vi "Edit_Template_File.vi"(0 "Mode":T3(ring), 7 "Template Filename":path, 11 "Data Filename":path) -> (6 "Template Filename Out":path)   [LabVIEW 2016]
uses:
  Anemometry/Anemometry Sub Vis/Data_plotting_vis/File_Template_Clus.ctl
  subVIs/Dispose_Channel.ctl
  Anemometry/Anemometry Sub Vis/Controls/Global_mode.ctl
panel:
  out "index of element":i32
  in  "Add New Channel Named":bool
  in  "Edit Maths Equation":bool
  out "Current Case Name":string
  in  "Organise Channels":bool
  in  "Add New Channels Fr File":bool
  in  "OK":bool
  in  "Search String":string
  in  "Listbox":i32(listbox)
  out "Channel Name":string
  in  "Cluster":T1 {"Tolerance" min=0.0 format="%#.4f"}
  # "> 20  or  <20  or  =hello   or \n£hello  (not equal to hello)"
  # "<<Characters_to_Match>>  <<Replace_Whole_String_with_this>>"
  # "<<Channel_Name>> contains <<Characters to match>> or\n<<Channel_Name>> does not contain <<Characters to match>>"
  # "<<Channel_Name_A>> + <<Channel_Name_B>> or\nConcatenate <<Channel_Name_A>> and <<Channel_Name_B>>"
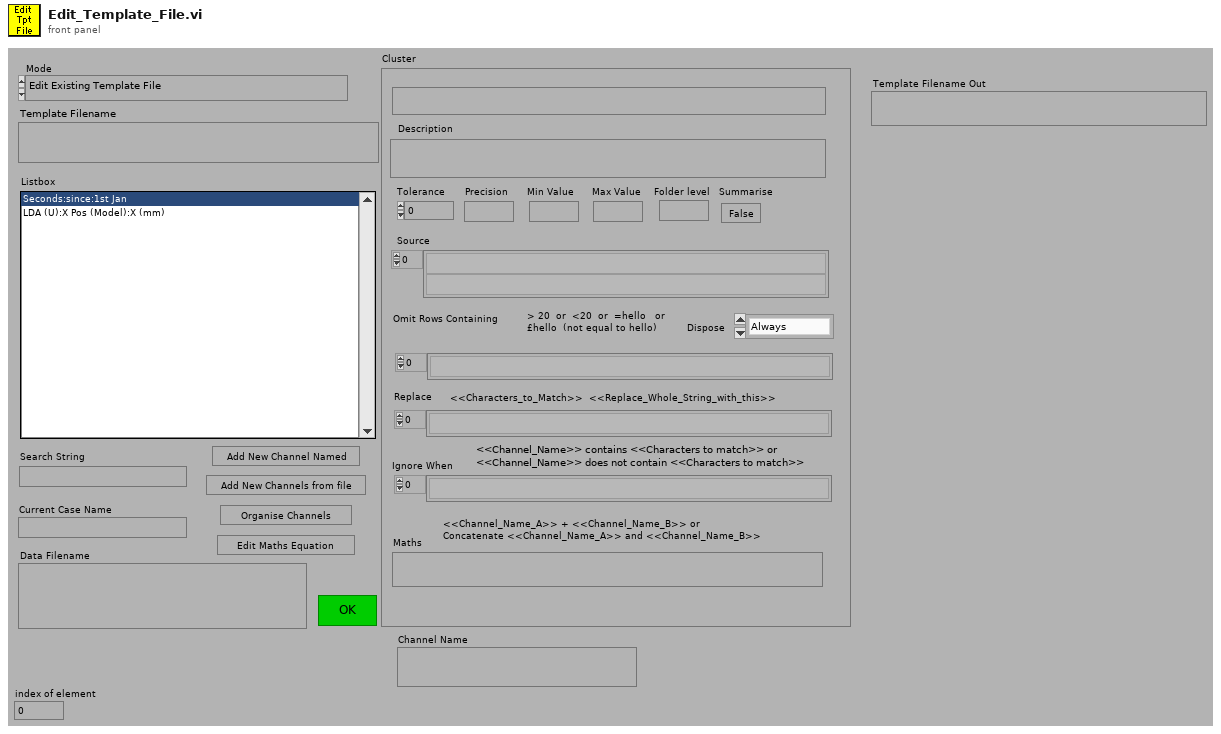
[diagram p1: front panel]
types:
  T1 = typedef "File_Template_Clus.ctl" = cluster{"Template Channel Name":string, "Description":string, "Tolerance":dbl, "Precision":string, "Folder level":string, "Source":string[], "Replace":string[], "Summarise":bool, "Min Value":string, "Maths":string, "Omit Rows Containing":string[], "Ignore When":string[], "Max Value":string, "Dispose":T2}
  T2 = typedef "Dispose_Channel.ctl" = enum16{"Always", "If Blank", "Never"}
  T3 = enum16{"Edit Existing Template File", "Create New Template File"}
  T4 = typedef "Global_mode.ctl" = enum16{"Read Global", "Load Global From File", "Write Global to File"}
  T5 = enum16{"Read Channels From File", "Read Channels from Server"}
  T6 = enum32{"existing file", "new file", "new or existing file", "existing dir", "new dir", "new or existing dir", "existing file (use LLBs)", "new file (use LLBs)", "new or existing file (use LLBs)", "new or existing file or directory (use LLBs)"}
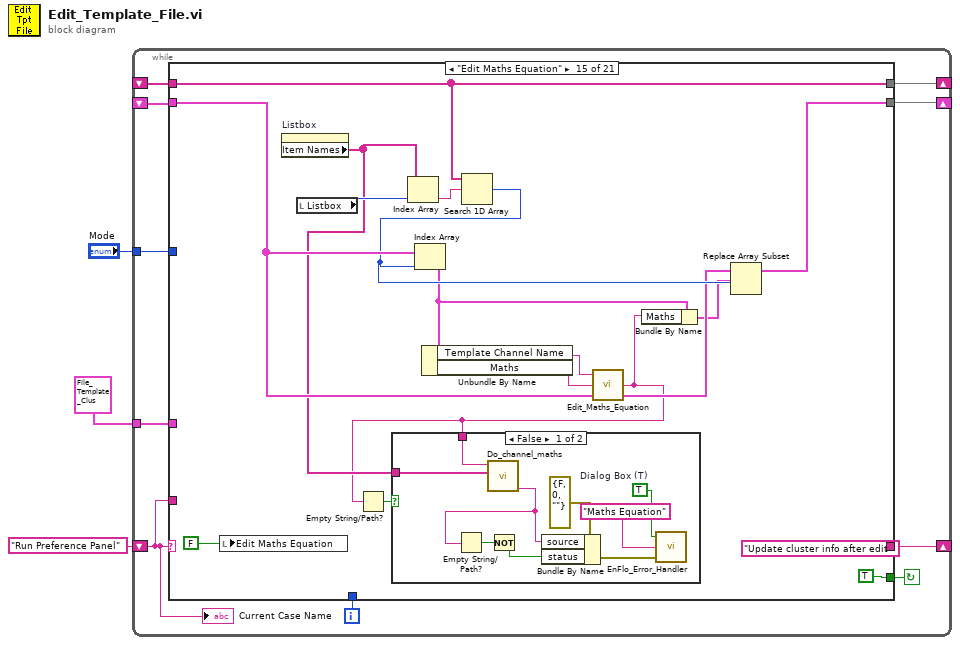
[diagram p0: block diagram]
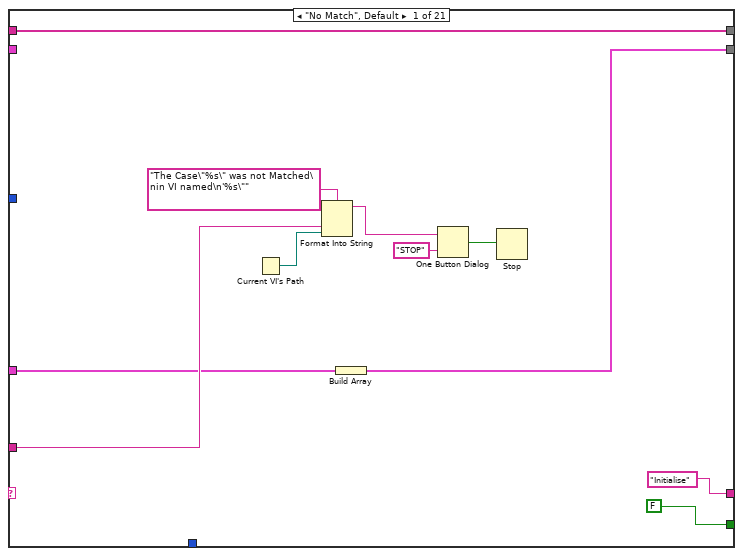
[diagram p2: hidden frame]
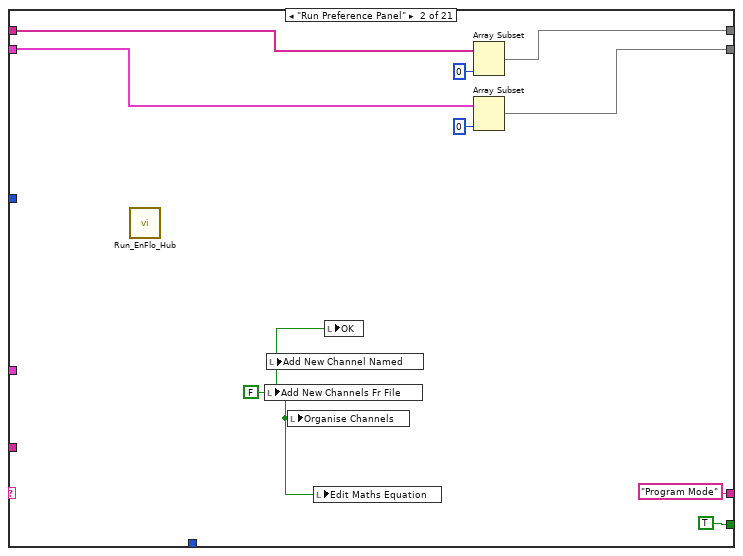
[diagram p3: hidden frame]
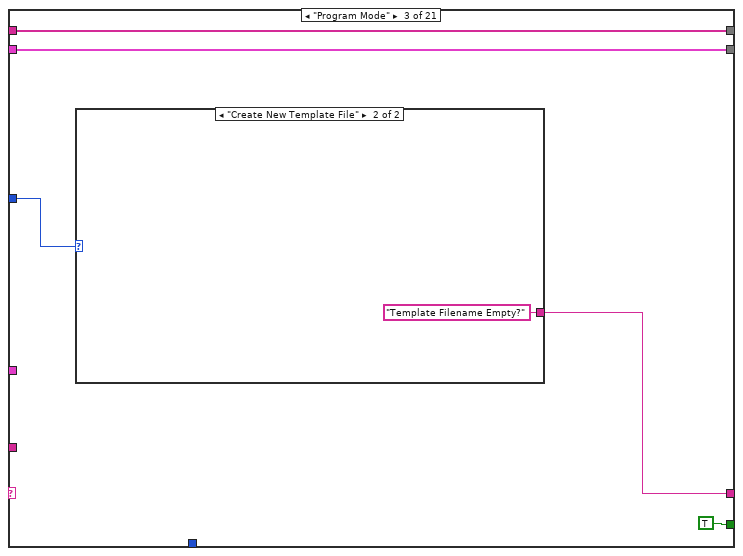
[diagram p4: hidden frame]
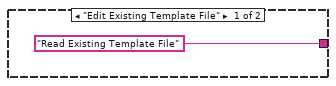
[diagram p5: hidden frame]
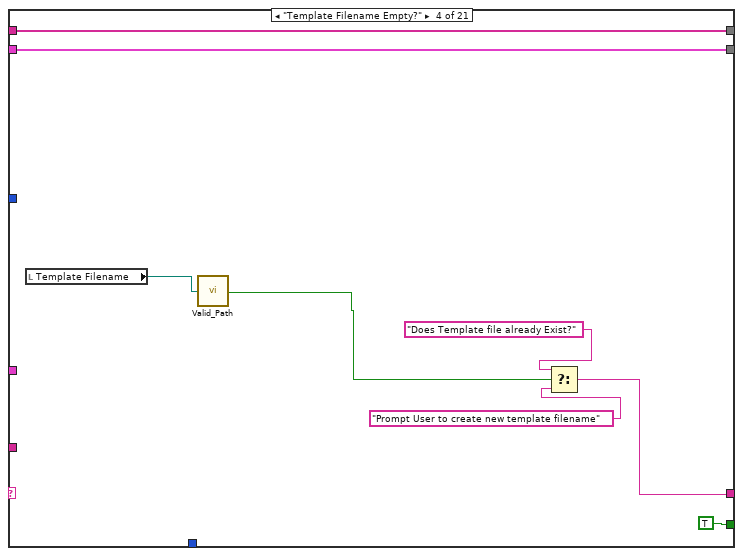
[diagram p6: hidden frame]
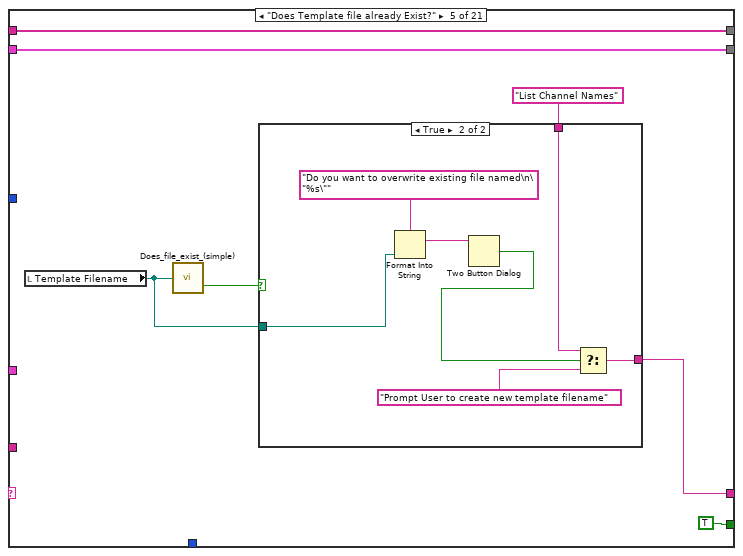
[diagram p7: hidden frame]
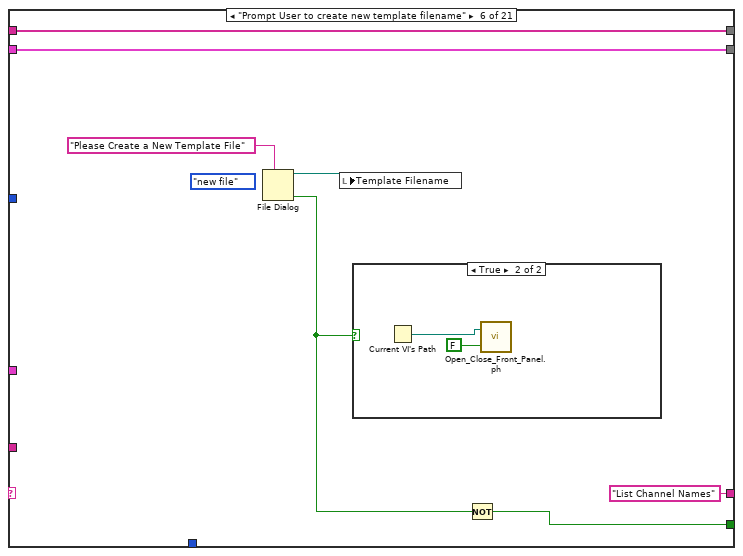
[diagram p9: hidden frame]
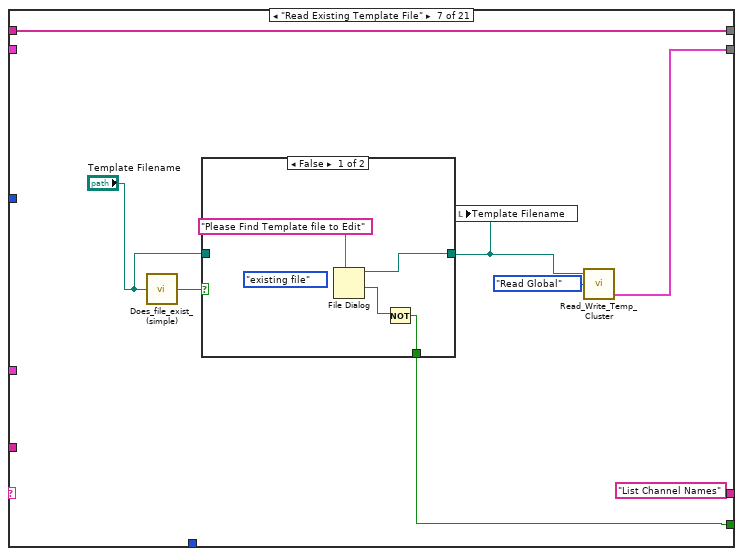
[diagram p11: hidden frame]
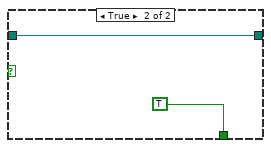
[diagram p12: hidden frame]
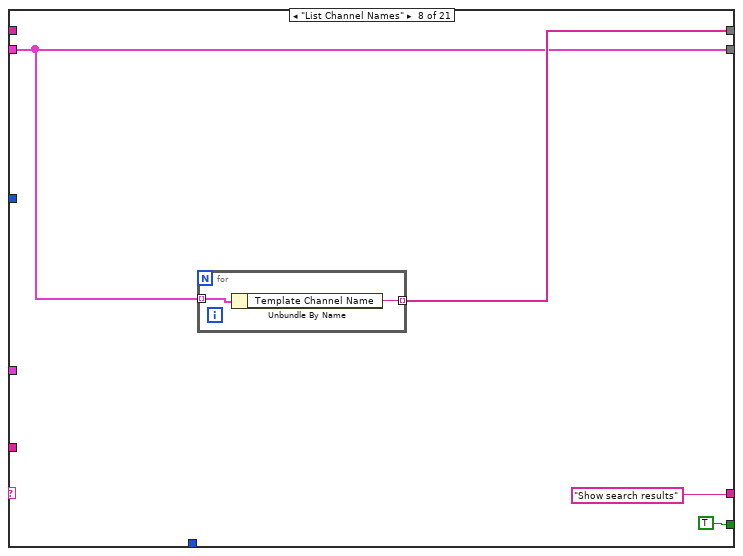
[diagram p13: hidden frame]
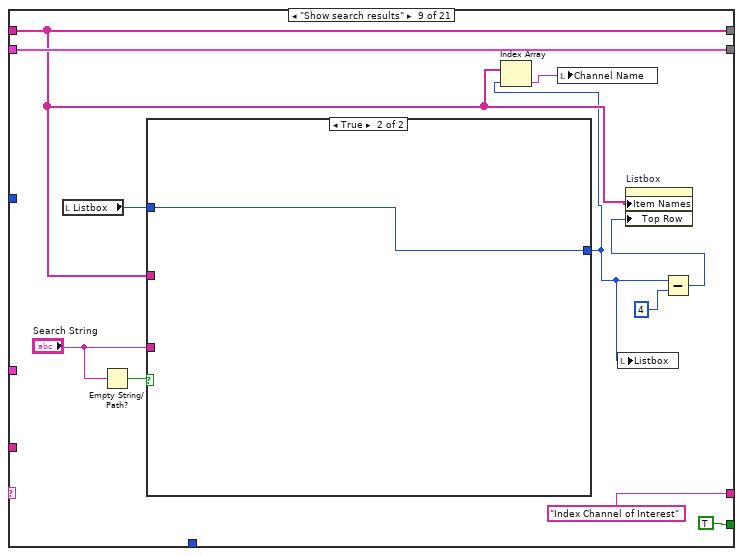
[diagram p14: hidden frame]
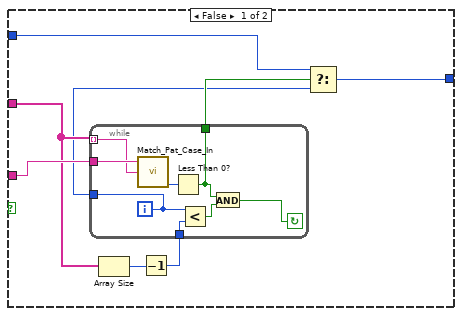
[diagram p15: hidden frame]
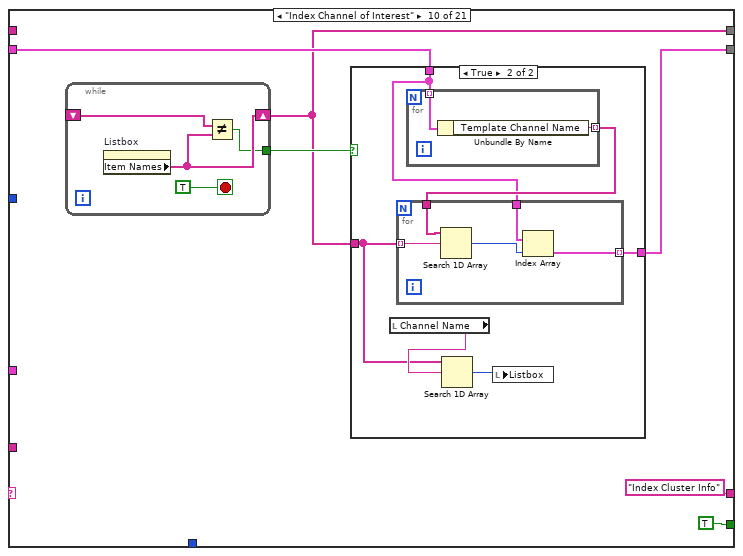
[diagram p16: hidden frame]
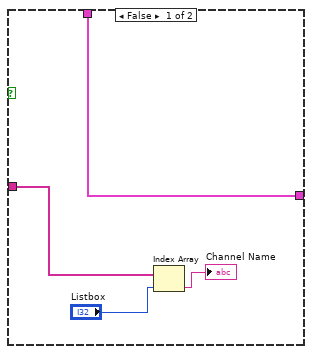
[diagram p17: hidden frame]
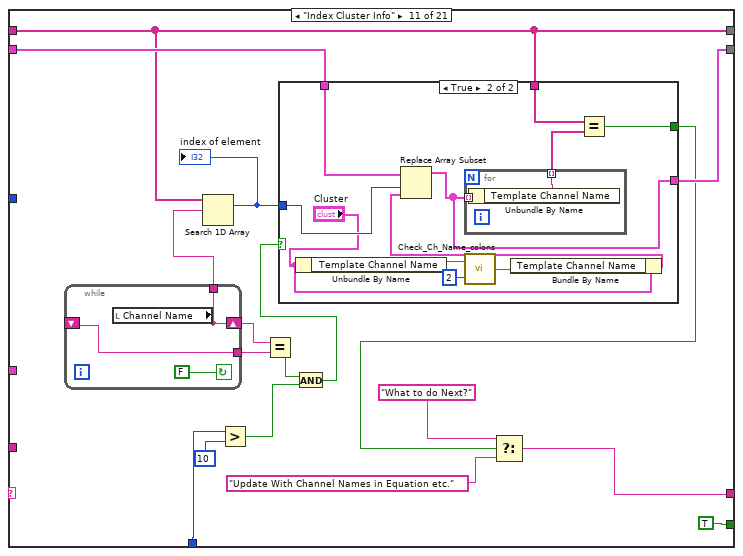
[diagram p18: hidden frame]
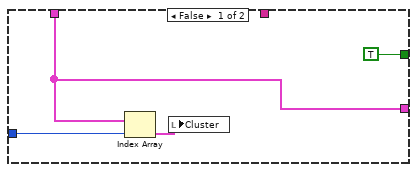
[diagram p19: hidden frame]
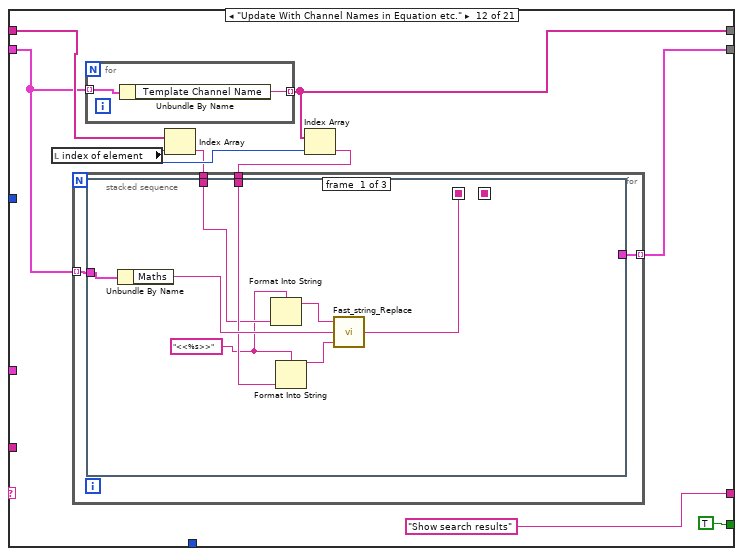
[diagram p20: hidden frame]
diagram:
  n1 = while {
    tunnel: T1 {"Template Channel Name"="", "Description"="", "Tolerance"=0.0, "Precision"="", "Folder level"="", "Source"=[], "Replace"=[], "Summarise"=FALSE, "Min Value"="", "Maths"="", "Omit Rows Containing"=[], "Ignore When"=[], "Max Value"="", "Dispose"=enum."Never"} ("Cluster") -> [w7]
    shift-left: _ -> [w8]
    shift-right: [w9] -> _
    tunnel: "Mode" -> [w11]
    shift-left: _ -> [w4]
    shift-right: [w10] -> _
    shift-left: "Run Preference Panel" -> [w6]
    shift-right: [w12] -> _
    i -> [w5]
    stop <- w13 continue-if-true
    n2 = case shown="\"Edit Maths Equation\"" w6 {
      tunnel: [FALSE TRUE TRUE TRUE TRUE w65 w73 TRUE TRUE TRUE TRUE TRUE TRUE TRUE TRUE TRUE TRUE TRUE TRUE TRUE FALSE] -> w13
      tunnel: ["Initialise" "Program Mode" w34 w45 w50 "List Channel Names" ("t") "List Channel Names" "Show search results" "Index Channel of Interest" "Index Cluster Info" w155 "Show search results" "Update cluster info after edit" "Update cluster info after edit" "Update cluster info after edit" "Save Template File" ("t") w333 w342 "Save Template File" w371 "End" ("t")] -> w12
      tunnel: w6 -> [w19 _ _ _ _ _ _ _ _ _ _ _ _ _ _ _ _ _ _ _ _]
      tunnel: w11 -> [_ _ w37 _ _ _ _ _ _ _ _ _ _ _ _ _ _ _ _ _ _]
      tunnel: [w14 w26 w35 w46 w53 w69 w76 w87 w99 w123 w158 w190 w228 w270 w287 w311 w336 w348 w362 w376 w383] -> w10
      tunnel: w4 -> [_ w27 w35 w46 w53 w69 _ w87 w99 w124 w162 w189 w230 w271 w292 w311 w336 w349 w368 w376 w383]
      tunnel: [w16 w29 w36 w47 w54 w70 w75 w89 w95 w121 w154 w191 w229 w272 w294 w313 w337 w350 w363 w375 w384] -> w9
      tunnel: w8 -> [w16 w30 w36 w47 w54 w70 w75 _ w95 _ w154 w192 w231 w273 w294 w313 w337 w350 w364 w375 w384]
      tunnel: w7 -> [w15 _ _ _ _ _ _ _ _ _ _ _ w227 _ _ _ _ _ w367 _ _]
      tunnel: w5 -> [_ _ _ _ _ _ _ _ _ _ w152 _ _ _ _ _ _ _ _ _ _]
      frame "No Match", Default {
        n3 = Current VI's Path() -> (path=w18:path)
        n4 = Format Into String(format string="The Case\"%s\" was not Matched\nin VI named\n'%s\"" ("Format String"), w19, w18) -> (resulting string=w22:string)  [unwired: 2 in, 1 out]
        n5 = Build Array(w15) -> (w14:T1[])
        n6 = One Button Dialog(message=w22, button name ("OK")="STOP") -> (true=w20:bool)
        n7 = Stop(stop? (T)=w20) -> ()
      }
      frame "Run Preference Panel" {
        w25 = FALSE ("Add channel Fr Results File")
        n8 = call "Run_EnFlo_Hub.vi"() -> ()  [unwired: 1 in, 7 out]
        n9 = local write "Add New Channels Fr File"(w25) -> ()
        n10 = local write "Add New Channel Named"(w25) -> ()
        n11 = local write "Organise Channels"(w25) -> ()
        n12 = local write "Edit Maths Equation"(w25) -> ()
        n13 = local write "OK"(w25) -> ()
        n14 = Array Subset(array=w30, length=0 ("Array Length")) -> (w29:string[])  [unwired: 1 in]
        n15 = Array Subset(array=w27, length=0 ("Array Length")) -> (w26:T1[])  [unwired: 1 in]
      }
      frame "Program Mode" {
        n16 = case shown="\"Create New Template File\"" w37 {
          tunnel: ["Read Existing Template File" "Template Filename Empty?"] -> w34
          frame "Edit Existing Template File" {
          }
          frame "Create New Template File" {
          }
        }
      }
      frame "Template Filename Empty?" {
        n17 = local read "Template Filename"() -> (w44:path)
        n18 = call "Valid_Path.vi"("Filename"=w44) -> ("Valid Path?"=w43:bool)
        n19 = Select(t="Does Template file already Exist?", s=w43, f="Prompt User to create new template filename" ("t")) -> (s? t:f=w45:string)
      }
      frame "Does Template file already Exist?" {
        n20 = local read "Template Filename"() -> (w51:path)
        n21 = call "Does_file_exist_(simple).vi"("Pathname"=w51) -> ("exists?"=w52:bool)
        n22 = case shown="True" w52 {
          tunnel: w51 -> [_ w63]
          tunnel: [w56 w58] -> w50
          tunnel: "List Channel Names" ("t") -> [w56 w57]
          frame False {
          }
          frame True {
            n23 = Format Into String(format string="Do you want to overwrite existing file named\n\"%s\"" ("Format String"), w63) -> (resulting string=w61:string)  [unwired: 2 in, 1 out]
            n24 = Two Button Dialog(message=w61) -> (T button?=w59:bool)  [unwired: 2 out]
            n25 = Select(t=w57, s=w59, f="Prompt User to create new template filename") -> (s? t:f=w58:string)
          }
        }
      }
      frame "Prompt User to create new template filename" {
        (unwired) T6."new file" ("select mode (2)")
        n26 = File Dialog(7:"Please Create a New Template File" ("prompt")) -> (1:w64:bool, 3:w68:path)  [unwired: 1 in, 7 out]
        n27 = local write "Template Filename"(w68) -> ()
        n28 = case shown="True" w64 {
          frame False {
          }
          frame True {
            n29 = Current VI's Path() -> (path=w72:path)
            n30 = call "Open_Close_Front_Panel.ph.vi"("Front Panel Window:Open"=FALSE, "VI path"=w72) -> ()  [unwired: 2 out]
          }
        }
        n31 = Not(x=w64) -> (.not. x?=w65:bool)
      }
      frame "Read Existing Template File" {
        n32 = call "Does_file_exist_(simple).vi"("Pathname"="Template Filename") -> ("exists?"=w79:bool)
        n33 = case shown="False" w79 {
          tunnel: [w84 w86] -> w74
          tunnel: "Template Filename" -> [_ w86]
          tunnel: [w81 TRUE] -> w73
          frame False {
            (unwired) T6."existing file" ("select mode (2)")
            n34 = File Dialog(7:"Please Find Template file to Edit" ("prompt")) -> (1:w82:bool, 3:w84:path)  [unwired: 1 in, 7 out]
            n35 = Not(x=w82) -> (.not. x?=w81:bool)
          }
          frame True {
          }
        }
        n36 = local write "Template Filename"(w74) -> ()
        n37 = call "Read_Write_Temp_Cluster.vi"("Mode"=Global_mode."Read Global", "Template File"=w74) -> ("Template Info Array Out"=w76:T1[])  [unwired: 1 in, 2 out]
      }
      frame "List Channel Names" {
        n38 = for {
          tunnel: w87 -> [w92] mode=indexing
          tunnel: [w91] -> w89 mode=indexing
          n39 = Unbundle By Name(w92) -> ("Template Channel Name"=w91:string)
        }
      }
      frame "Show search results" {
        n40 = local read "Listbox"() -> (w94:i32)
        n41 = Empty String/Path?(string/path="Search String") -> (empty?=w101:bool)
        n42 = case shown="True" w101 {
          tunnel: "Search String" -> [w111 _]
          tunnel: w95 -> [w110 _]
          tunnel: w94 -> [w106 w120]
          tunnel: [w104 w120] -> w93
          frame False {
            n43 = Array Size(array=w110) -> (size(s)=w109:i32)
            n44 = Decrement(x=w109) -> (x-1=w108:i32)
            n45 = while {
              tunnel: w111 -> [w119]
              tunnel: w110 -> [w118] mode=indexing
              tunnel: w108 -> [w116]
              tunnel: [w113] -> w107
              tunnel: [w112] -> w105
              i -> [w112]
              stop <- w114 continue-if-true
              n46 = call "Match_Pat_Case_In.vi"("String to match"=w119, "String"=w118) -> ("offset past match"=w117:i32)  [unwired: 1 in, 3 out]
              n47 = Less Than 0?(x=w117) -> (x < 0?=w113:bool)
              n48 = Less?(x=w112, y=w116) -> (x < y?=w115:bool)
              n49 = And(x=w113, y=w115) -> (x .and. y?=w114:bool)
            }
            n50 = Select(t=w106, s=w107, f=w105) -> (s? t:f=w104:i32)
          }
          frame True {
          }
        }
        n51 = Index Array(array=w95, index=w93) -> (element=w96:string)
        n52 = local write "Channel Name"(w96) -> ()
        n53 = local write "Listbox"(w93) -> ()
        n54 = Subtract(x=w93, y=4) -> (x-y=w97:i32)
        n55 = property on="Listbox" class="LstBox (strict)"("Item Names"=w95, "Top Row"=w97) -> ()  [unwired: 2 in, 2 out]
      }
      frame "Index Channel of Interest" {
        n56 = while {
          shift-right: [w146] -> w121
          shift-left: _ -> [w147]
          tunnel: [w144] -> w122
          stop <- TRUE stop-if-true
          n57 = property on="Listbox" class="LstBox (strict)"() -> ("Item Names"=w146:string[])  [unwired: 2 in, 2 out]
          n58 = Not Equal?(x=w147, y=w146) -> (x != y?=w144:bool)
        }
        n59 = case shown="True" w122 {
          tunnel: w121 -> [w128 w132]
          tunnel: w124 -> [w130 w135]
          tunnel: [w130 w134] -> w123
          frame False {
            n60 = Index Array(array=w128, index="Listbox") -> (element=→"Channel Name":string)
          }
          frame True {
            n61 = local read "Channel Name"() -> (w133:string)
            n62 = for {
              tunnel: w135 -> [w143] mode=indexing
              tunnel: [w142] -> w136 mode=indexing
              n63 = Unbundle By Name(w143) -> ("Template Channel Name"=w142:string)
            }
            n64 = for {
              tunnel: w136 -> [w141]
              tunnel: w132 -> [w140] mode=indexing
              tunnel: w135 -> [w138]
              tunnel: [w137] -> w134 mode=indexing
              n65 = Search 1D Array(1D array=w141, element=w140) -> (index of element=w139:i32)  [unwired: 1 out]
              n66 = Index Array(array=w138, index=w139) -> (element=w137:T1)
            }
            n67 = Search 1D Array(1D array=w132, element=w133) -> (index of element=w131:i32)  [unwired: 1 out]
            n68 = local write "Listbox"(w131) -> ()
          }
        }
      }
      frame "Index Cluster Info" {
        n69 = while {
          tunnel: [w166] -> w159
          tunnel: [w167] -> w160
          shift-left: _ -> [w167]
          shift-right: [w166] -> w161
          stop <- FALSE continue-if-true
          n70 = local read "Channel Name"() -> (w166:string)
        }
        n71 = Search 1D Array(1D array=w154, element=w159) -> (index of element=w163:i32)  [unwired: 1 out]
        "index of element" <- w163
        n72 = Greater?(x=w152, y=10) -> (0:w149:bool)
        n73 = Equal?(x=w161, y=w160) -> (x = y?=w150:bool)
        n74 = And(x=w150, y=w149) -> (x .and. y?=w148:bool)
        n75 = case shown="True" w148 {
          tunnel: w163 -> [w171 w181]
          tunnel: w162 -> [w169 w182]
          tunnel: [w169 w178] -> w158
          tunnel: w154 -> [_ w179]
          tunnel: [TRUE w177] -> w153
          frame False {
            n76 = Index Array(array=w169, index=w171) -> (element=w170:T1)
            n77 = local write "Cluster"(w170) -> ()
          }
          frame True {
            n78 = Unbundle By Name("Cluster") -> ("Template Channel Name"=w175:string)
            n79 = call "Check_Ch_Name_colons.vi"("No of Colons"=2, "Ch Name in"=w175) -> ("Ch Name out"=w174:string)
            n80 = Bundle By Name(cluster="Cluster", "Template Channel Name"=w174) -> (w172:T1)
            n81 = Replace Array Subset(array=w182, new element=w172, index=w181) -> (w178:T1[])
            n82 = for {
              tunnel: w178 -> [w184] mode=indexing
              tunnel: [w183] -> w180 mode=indexing
              n83 = Unbundle By Name(w184) -> ("Template Channel Name"=w183:string)
            }
            n84 = Equal?(x=w179, y=w180) -> (x = y?=w177:bool)
          }
        }
        n85 = Select(t="What to do Next?", s=w153, f="Update With Channel Names in Equation etc.") -> (s? t:f=w155:string)
      }
      frame "Update With Channel Names in Equation etc." {
        n86 = local read "index of element"() -> (w187:i32)
        n87 = for {
          tunnel: w189 -> [w224] mode=indexing
          tunnel: [w223] -> w191 mode=indexing
          n88 = Unbundle By Name(w224) -> ("Template Channel Name"=w223:string)
        }
        n89 = Index Array(array=w192, index=w187) -> (element=w186:string)
        n90 = Index Array(array=w191, index=w187) -> (element=w185:string)
        n91 = for {
          tunnel: w189 -> [w195] mode=indexing
          tunnel: w185 -> [w197]
          tunnel: [w194] -> w190 mode=indexing
          tunnel: w186 -> [w196]
          n92 = stacked-sequence {
            seq-local: [w199 _ _] -> [_ _ w222]
            seq-local: [_ w207 _] -> [_ _ w220]
            tunnel: w195 -> [w205 w211 w219]
            tunnel: w197 -> [w203 w209 _]
            tunnel: w196 -> [w200 w208 _]
            tunnel: [_ _ w221] -> w194
            frame #0 {
              w198 = "<<%s>>" ("Format String")
              n93 = Unbundle By Name(w205) -> ("Maths"=w204:string)
              n94 = Format Into String(format string=w198, w200) -> (resulting string=w201:string)  [unwired: 2 in, 1 out]
              n95 = Format Into String(format string=w198, w203) -> (resulting string=w202:string)  [unwired: 2 in, 1 out]
              n96 = call "Fast_string_Replace.vi"("Replace match with:"=w202, "Input String"=w204, "regular expression"=w201) -> ("Output String"=w199:string)  [unwired: 2 out]
            }
            frame #1 {
              n97 = Unbundle By Name(w211) -> ("Ignore When"=w210:string[])
              n98 = for {
                tunnel: w210 -> [w218] mode=indexing
                tunnel: w209 -> [w217]
                tunnel: w208 -> [w214]
                tunnel: [w213] -> w207 mode=indexing
                tunnel: "<<%s>>" ("Format String") -> [w212]
                n99 = Format Into String(format string=w212, w214) -> (resulting string=w215:string)  [unwired: 2 in, 1 out]
                n100 = Format Into String(format string=w212, w217) -> (resulting string=w216:string)  [unwired: 2 in, 1 out]
                n101 = call "Fast_string_Replace.vi"("Replace match with:"=w216, "Input String"=w218, "regular expression"=w215) -> ("Output String"=w213:string)  [unwired: 2 out]
              }
            }
            frame #2 {
              n102 = Bundle By Name(cluster=w219, "Maths"=w222, "Ignore When"=w220) -> (w221:T1)
            }
          }
        }
      }
      frame "Select New Channel" {
        n103 = local read "Add New Channel Named"() -> (w226:bool)
        n104 = case shown="False" w226 {
          tunnel: [w236 w242] -> w232
          tunnel: [FALSE ("Add channel Fr Results File") FALSE ("Add channel Fr Results File")] -> w225
          frame False {
            n105 = call "Select_a_Channel.vi"("Mode"=T5."Read Channels From File", "Data Filename"="Data Filename") -> ("Selected Channel Names"=w236:string[], "Data Filename Out"=w238:path)  [unwired: 1 in, 4 out]
            n106 = local write "Data Filename"(w238) -> ()
          }
          frame True {
            n107 = call "Input_String_Dialog.vi"("Message to user"="Enter New Channel Name") -> ("Ok Out"=w244:bool, "Output string"=w245:string)  [unwired: 1 in]
            n108 = Build Array(w245) -> (w243:string[])
            n109 = Select(t=w243, s=w244, f=string[] []) -> (s? t:f=w242:string[])
          }
        }
        n110 = for {
          tunnel: w232 -> [w251] mode=indexing
          shift-right: [w249] -> w229
          shift-left: w231 -> [w250]
          shift-right: [w252] -> w228
          shift-left: w230 -> [w253]
          tunnel: w227 -> [w255]
          n111 = Build Array(w251) -> (w258:string[])
          n112 = while {
            tunnel: [w259] -> w248
            tunnel: w251 -> [w261]
            tunnel: w250 -> [w262]
            i -> [w260]
            stop <- w263 continue-if-true
            n113 = case shown="1, Default" w260 {
              tunnel: w260 -> [_ w266]
              tunnel: [w265 w268] -> w259
              tunnel: w261 -> [w265 w267]
              frame 0 {
              }
              frame 1, Default {
                n114 = Format Into String(format string="%s_DUPLICATE%d" ("Format String"), w267, w266) -> (resulting string=w268:string)  [unwired: 2 in, 1 out]
              }
            }
            n115 = Search 1D Array(1D array=w262, element=w259) -> (index of element=w264:i32)  [unwired: 1 out]
            n116 = Greater Or Equal To 0?(x=w264) -> (x >= 0?=w263:bool)
          }
          n117 = Bundle By Name(cluster=w255, "Template Channel Name"=w248, "Source"=w258, "Summarise"=TRUE ("Bundle Element"), "Dispose"=Dispose_Channel."Never", "Tolerance"=1.0 ("Bundle Element")) -> (w254:T1)
          n118 = Build Array (concatenate)(w253, w254) -> (w252:T1[])
          n119 = Build Array (concatenate)(w250, w248) -> (w249:string[])
        }
        n120 = local write "Add New Channel Named"(w225) -> ()
        n121 = local write "Add New Channels Fr File"(w225) -> ()
      }
      frame "Organise Channels" {
        n122 = call "Organise_String_Array.vi"("Input Array"=w273) -> ("Output Array"=w272:string[])
        n123 = for {
          tunnel: w273 -> [w281]
          tunnel: w272 -> [w280] mode=indexing
          tunnel: w271 -> [w278]
          tunnel: [w277] -> w270 mode=indexing
          n124 = Search 1D Array(1D array=w281, element=w280) -> (index of element=w279:i32)  [unwired: 1 out]
          n125 = Index Array(array=w278, index=w279) -> (element=w277:T1)
        }
        n126 = local write "Organise Channels"(FALSE ("Add channel Fr Results File")) -> ()
      }
      frame "Edit Maths Equation" {
        n127 = local write "Edit Maths Equation"(FALSE ("Add channel Fr Results File")) -> ()
        n128 = property on="Listbox" class="LstBox (strict)"() -> ("Item Names"=w284:string[])  [unwired: 2 in, 2 out]
        n129 = local read "Listbox"() -> (w295:i32)
        n130 = Index Array(array=w284, index=w295) -> (element=w293:string)
        n131 = Search 1D Array(1D array=w294, element=w293) -> (index of element=w289:i32)  [unwired: 1 out]
        n132 = Index Array(array=w292, index=w289) -> (element=w288:T1)
        n133 = Unbundle By Name(w288) -> ("Template Channel Name"=w291:string, "Maths"=w290:string)
        n134 = call "Edit_Maths_Equation.vi"("Template Info Array"=w292, "Maths Equation In"=w290, "Channel Name"=w291) -> ("Template Info Array Out"=w286:T1[], "Maths Equation Out"=w283:string)  [unwired: 1 out]
        n135 = Empty String/Path?(string/path=w283) -> (empty?=w282:bool)
        n136 = case shown="False" w282 {
          tunnel: w284 -> [w300 _]
          tunnel: w283 -> [w299 _]
          frame False {
            w301 = TRUE  # Dialog Box (T)
            n137 = call "Do_channel_maths.vi"("Channel Names"=w300, "Maths Equation"=w299) -> ("Error String"=w305:string)  [unwired: 2 in, 3 out]
            n138 = Empty String/Path?(string/path=w305) -> (empty?=w307:bool)
            n139 = Not(x=w307) -> (.not. x?=w304:bool)
            n140 = Bundle By Name(cluster=errorcluster {"status"=FALSE, "code"=0, "source"=""} ("error in (no error)"), "source"=w305, "status"=w304) -> (w303:errorcluster)
            n141 = call "EnFlo_Error_Handler.vi"("error in (no error)"=w303, "Error Type"="Maths Equation", "Dialog Box (T)"=w301) -> ()  [unwired: 3 out]
          }
          frame True {
          }
        }
        n142 = Bundle By Name(cluster=w288, "Maths"=w283) -> (w285:T1)
        n143 = Replace Array Subset(array=w286, new element=w285, index=w289) -> (w287:T1[])
      }
      frame "Update cluster info after edit" {
        n144 = local read "Channel Name"() -> (w309:string)
        n145 = Search 1D Array(1D array=w313, element=w309) -> (index of element=w312:i32)  [unwired: 1 out]
        n146 = Index Array(array=w311, index=w312) -> (element=w310:T1)
        n147 = local write "Cluster"(w310) -> ()
      }
      frame "What to do Next?" {
        n148 = while {
          tunnel: [w340] -> w331
          shift-left: _ -> [w340]
          shift-right: [w341] -> w332
          stop <- FALSE continue-if-true
          n149 = local read "Search String"() -> (w341:string)
        }
        n150 = Not Equal?(x=w332, y=w331) -> (x != y?=w328:bool)
        n151 = Select(t="List Channel Names", s=w328, f="Index Channel of Interest") -> (s? t:f=w325:string)
        n152 = Select(t="Select New Channel", s="Add New Channels Fr File", f=w325) -> (s? t:f=w322:string)
        n153 = Select(t="Organise Channels", s="Organise Channels", f=w322) -> (s? t:f=w315:string)
        n154 = Select(t="Edit Maths Equation", s="Edit Maths Equation", f=w315) -> (s? t:f=w317:string)
        n155 = Select(t="Select New Channel", s="Add New Channel Named", f=w317) -> (s? t:f=w316:string)
        n156 = Select(t="Check Template File", s="OK", f=w316) -> (s? t:f=w333:string)
      }
      frame "Check Template File" {
        n157 = for {
          tunnel: w349 -> [w355] mode=indexing
          tunnel: [w354] -> w348 mode=indexing
          tunnel: [w351] -> w346 mode=indexing
          n158 = Unbundle By Name(w355) -> ("Template Channel Name"=w356:string)
          n159 = call "Check_Ch_Name_colons.vi"("No of Colons"=2, "Ch Name in"=w356) -> ("Ch Name out"=w353:string)
          n160 = Bundle By Name(cluster=w355, "Template Channel Name"=w353) -> (w354:T1)
          n161 = Equal?(x=w353, y="Raw:Data:Filename") -> (x = y?=w351:bool)
        }
        n162 = Or Array Elements(Boolean array=w346) -> (logical OR=w343:bool)
        n163 = Select(t="Save Template File", s=w343, f="Add Raw Data Filename") -> (s? t:f=w342:string)
      }
      frame "Add Raw Data Filename" {
        w365 = "Raw:Data:Filename" ("y")
        n164 = Bundle By Name(cluster=w367, "Template Channel Name"=w365, "Dispose"=Dispose_Channel."Never", "Summarise"=TRUE) -> (w366:T1)
        n165 = Build Array (concatenate)(w368, w366) -> (w362:T1[])
        n166 = Build Array (concatenate)(w364, w365) -> (w363:string[])
      }
      frame "Save Template File" {
        n167 = local write "Mode"(T3."Edit Existing Template File" ("Mode")) -> ()
        n168 = local read "Template Filename"() -> (w377:path)
        "Template Filename Out" <- w377
        n169 = call "Read_Write_Temp_Cluster.vi"("Template Info Array"=w376, "Mode"=Global_mode."Write Global to File", "Template File"=w377) -> ()  [unwired: 3 out]
        n170 = local read "OK"() -> (w374:bool)
        n171 = Select(t="Close Panel", s=w374, f="List Channel Names") -> (s? t:f=w371:string)
      }
      frame "Close Panel" {
        n172 = Current VI's Path() -> (path=w380:path)
        n173 = call "Open_Close_Front_Panel.ph.vi"("Front Panel Window:Open"=FALSE, "VI path"=w380) -> ()  [unwired: 2 out]
      }
    }
    "Current Case Name" <- w6
  }
